vi "FestoCPX.Global.Init.vi"(8 "error in (no error)":errorcluster) -> (0 "error out":errorcluster)   [LabVIEW 2015]
uses:
  FestoCPX.DO.Data.Fglb.Action.ctl
  FestoCPX.DI.Data.Fglb.Action.ctl
  FestoCPX.Global.vi
  Global/ApplicationGlobal.vi
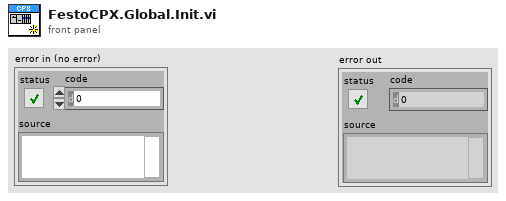
[diagram p1: front panel]
types:
  T1 = typedef "FestoCPX.DI.Data.Fglb.Action.ctl" = enum16{"init", "setup", "set", "simul", "get"}
  T2 = typedef "FestoCPX.DO.Data.Fglb.Action.ctl" = enum16{"init", "set", "get", "check", "select", "reset"}
  T3 = typedef "FestoCPX.Data.Sets.ctl" = cluster{"IP":string, "Timeout":i32, "Config.DI":T4[], "Config.DO":T6[]}
  T4 = typedef "FestoCPX.DI.Sets.ctl" = cluster{"Name":string, "Channel":T5, "Negate":bool}
  T5 = typedef "FestoCPX.DI.ctl" = enum16{"1.0", "1.1", "1.2", "1.3", "1.4", "1.5", "1.6", "1.7", "2.0", "2.1", "2.2", "2.3", "2.4", "2.5", "2.6", "2.7", "3.0", "3.1", "3.2", "3.3", "3.4", "3.5", "3.6", "3.7", "4.0", "4.1", "4.2", "4.3", "4.4", "4.5", "4.6", "4.7", "5.0", "5.1", "5.2", "5.3", "5.4", "5.5", "5.6", "5.7"}
  T6 = typedef "FestoCPX.DO.Sets.ctl" = cluster{"Name":string, "Channel":T7, "Negate":bool, "Default":bool}
  T7 = typedef "FestoCPX.DO.ctl" = enum16{"1.0", "1.1", "1.2", "1.3", "1.4", "1.5", "1.6", "1.7", "2.0", "2.1", "2.2", "2.3", "2.4", "2.5", "2.6", "2.7", "Q4K1", "Q4K2", "Q5K1", "Q5K2", "Q6K1", "Q6K2", "Q7K1", "Q7K2", "Q8K1", "Q8K2", "Q9K1", "Q9K2", "Q10K1", "Q10K2", "Q11K1", "Q11K2", "Q12K1", "Q12K2", "Q13K1", "Q13K2"}
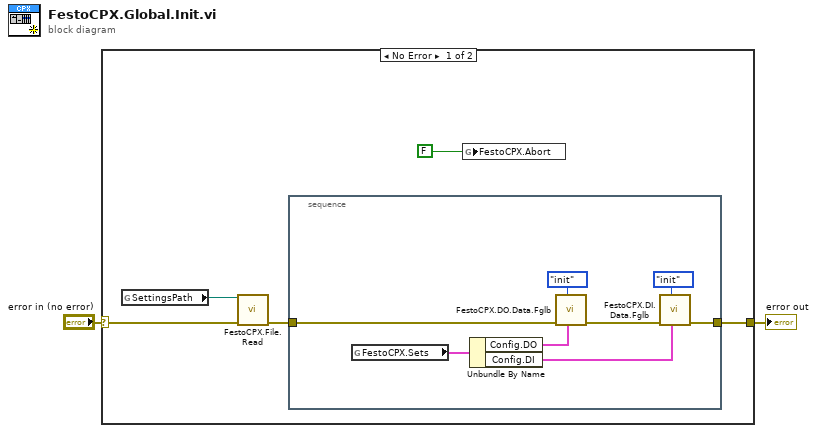
[diagram p0: block diagram]
diagram:
  n1 = case shown="No Error" "error in (no error)" {
    selector: "error in (no error)" -> [w7 w16]
    tunnel: [w4 w16] -> w1
    frame No Error {
      n2 = global read "ApplicationGlobal.vi" "SettingsPath"() -> (w6:path)
      n3 = call "FestoCPX.File.Read.vi"("error in"=w7, "Settings dir"=w6) -> ("error out"=w5:errorcluster)  [unwired: 9 in]
      n4 = stacked-sequence {
        tunnel: w5 -> [w14]
        tunnel: [w12] -> w4
        frame #0 {
          n5 = global read "FestoCPX.Global.vi" "FestoCPX.Sets"() -> (w11:T3)
          n6 = Unbundle By Name(w11) -> ("Config.DO"=w9:T6[], "Config.DI"=w10:T4[])
          n7 = call "FestoCPX.DO.Data.Fglb.vi"("Config"=w9, "state (get all)"=FestoCPX.DO.Data.Fglb.Action."init", "error in (no error)"=w14) -> ("error out"=w8:errorcluster)  [unwired: 6 in, 2 out]
          n8 = call "FestoCPX.DI.Data.Fglb.vi"("Config"=w10, "state (get)"=FestoCPX.DI.Data.Fglb.Action."init", "error in (no error)"=w8) -> ("error out"=w12:errorcluster)  [unwired: 7 in, 1 out]
        }
      }
      n9 = global write "FestoCPX.Global.vi" "FestoCPX.Abort"(FALSE ("CAN.Abort")) -> ()
    }
    frame Error {
    }
  }
  "error out" <- w1
